vi "AuMT8852B EDR Differential Phase Encoding Configuration.vi"(5 "Settings":T1={"Low frequency selection"=enum."Use low frequency", "Medium frequency selection"=enum."Use medium frequency", "High frequency selection"=enum."Use high frequency", "Low TX frequency"=2480.0, "Medium TX frequency"=2402.0, "High TX frequency"=2402.0, "Percentage of packets limit"=99.0, "2DHx test packet"=enum."OFF", "3DHx test packet"=enum."OFF", "Hop selection"=enum."Test with hopping off and on", "Number of packets"=100} {"Percentage of packets limit" format="%.2f"}, 7 "Set/Get (Set)":enum16{"Set", "Get"}(ring), 8 "error in (no error)":errorcluster, 10 "Script (3)":i32=3, 11 "VISA session":refnum<visa-resource-name>) -> (0 "error out":errorcluster, 2 "error code":i32, 3 "VISA session out":refnum<visa-resource-name>, 4 "Settings out":T1={"Low frequency selection"=enum."Use low frequency", "Medium frequency selection"=enum."Use medium frequency", "High frequency selection"=enum."Use high frequency", "Low TX frequency"=2480.0, "Medium TX frequency"=2402.0, "High TX frequency"=2402.0, "Percentage of packets limit"=100.0, "2DHx test packet"=enum."OFF", "3DHx test packet"=enum."OFF", "Hop selection"=enum."Test with hopping off and on", "Number of packets"=7408} {"Percentage of packets limit" format="%.2f"})   [LabVIEW 2017]
doc: "Anritsu MT8852B Bluetooth Tester\n\nConfigures the instrument for the EDR Differential Phase Encoding test.\n\nINPUTS\nSet/Get - whether the values are being sent to or retrieved from the instrument.\nScript - which of the stored scripts (1-10) will be queried or configured. Scripts 1 and 2 are read-only.\nSettings - parameters of the test to be written.\n\nOUTPUTS\nSettings out - current parameters of the test."
uses:
  <instrlib>/aumt8852B/General/Utilities/MT8850 Test Parameters.ctl
  <instrlib>/aumt8852B/General/Utilities/MT8850 Frequency Units.ctl
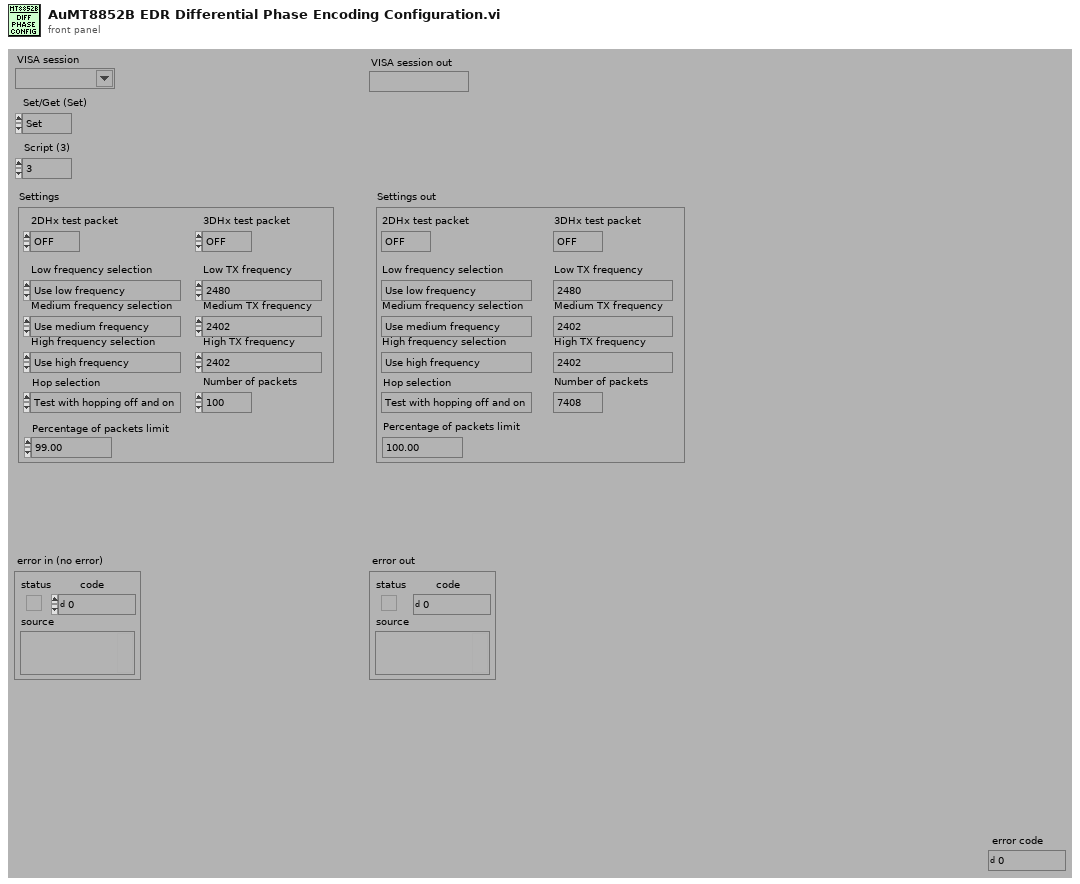
[diagram p1: front panel]
types:
  T1 = cluster{"Low frequency selection":enum16{"Don't use low frequency", "Use low frequency"}, "Medium frequency selection":enum16{"Don't use medium frequency", "Use medium frequency"}, "High frequency selection":enum16{"Don't use high frequency", "Use high frequency"}, "Low TX frequency":dbl, "Medium TX frequency":dbl, "High TX frequency":dbl, "Percentage of packets limit":dbl, "2DHx test packet":enum16{"OFF", "Longest", "2-DH1", "2-DH3", "2-DH5"}, "3DHx test packet":enum16{"OFF", "Longest", "3-DH1", "3-DH3", "3-DH5"}, "Hop selection":enum16{"Test with hopping on", "Test with hopping off", "Test with hopping off and on"}, "Number of packets":i32}
  T2 = enum16{"Output power", "Power control", "Modulation characteristics", "Initial carrier", "Carrier drift", "Single slot sensitivity", "Multiple slot sensitivity", "Maximum input power", "EDR Relative transmit power", "EDR Carrier frequency and stability", "EDR Differential phase encoding", "EDR Sensitivity", "EDR BER floor sensitivity", "EDR Maximum input power"}
  T3 = typedef "MT8850 Frequency Units.ctl" = enum16{"Channel", "Hz", "kHz", "MHz", "GHz"}
  T4 = typedef "MT8850 Test Parameters.ctl" = enum16{"Use low frequency", "Use medium frequency", "Use high frequency", "Low TX frequency", "Low RX frquency", "Medium TX frequency", "Medium RX frequency", "High TX frequency", "High RX frequency", "Number of packets", "Average high limit", "Average low limit", "Peak power limit", "Max power step limit", "Min power step limit", "f1 average minimum", "f1 average maximum", "f2 maximum", "f1/f2 average maximum", "Hop selection", "Use DH1 packets", "Use DH3 packets", "Use DH5 packets", "1 slot packet drift limit", "3 slot packet drift limit", "5 slot packet drift limit", "Drift rate limit", "TX power level", "Frequency offset", "Symbol timing", "Modulation index", "BER limit", "FER limit", "Use averaging high limit", "Use averaging low limit", "Use peak power limit", "Packet type", "Test control", "Use max power step limit", "Use min power step limit", "Number of cycles", "Use f1 average maximum", "Use f1 average minimum", "Use f2 maximum", "Use f1/f2 average maximum", "Hop mode", "Maximum negative limit", "Maximum positive limit", "Use maximum negative limit", "Use maximum positive limit", "Use 1 slot packet drift limit", "Use 3 slot packet drift limit", "Use 5 slot packet drift limit", "Use drift rate limit", "Use BER limit", "Use FER limit", "Use dirty parameter table", "Use null packet drift limit", "Null packet drift limit", "Minimum power", "Power delay", "Packet count", "Payload toggle", "Output power level", "2DHX packet type", "3DHX packet type", "Number of blocks", "TX and RX low frequency", "TX and RX medium frequency", "TX and RX high frequency", "TX frequency", "RX frequency", "Threshold bit count", "Total test bit count", "Number of bits", "PDPSK to PGFSK lower limit", "PDPSK to PGFSK upper limit", "Initial frequency error upper limit", "Initial frequency error lower limit", "Frequency error upper limit", "Frequency error lower limit", "Block frequency error upper limit", "Block frequency error lower limit", "2Mbs RMS DEVM limit", "3Mbs RMS DEVM limit", "2Mbs Peak DEVM limit", "3Mbs Peak DEVM limit", "2Mbs 99% packets DEVM limit", "3Mbs 99% packets DEVM limit", "Percentage of no error packets limit", "Threshold error limit", "Total test error limit"}
  T5 = enum16{"Simulate", "Range check", "Cache", "Query instrument status"}
  T6 = enum16{"Test with hopping on", "Test with hopping off", "Test with hopping off and on"}
  T7 = enum16{"OFF", "Longest", "3-DH1", "3-DH3", "3-DH5"}
  T8 = enum16{"OFF", "Longest", "2-DH1", "2-DH3", "2-DH5"}
  T9 = enum16{"Don't use high frequency", "Use high frequency"}
  T10 = enum16{"Don't use medium frequency", "Use medium frequency"}
  T11 = enum16{"Don't use low frequency", "Use low frequency"}
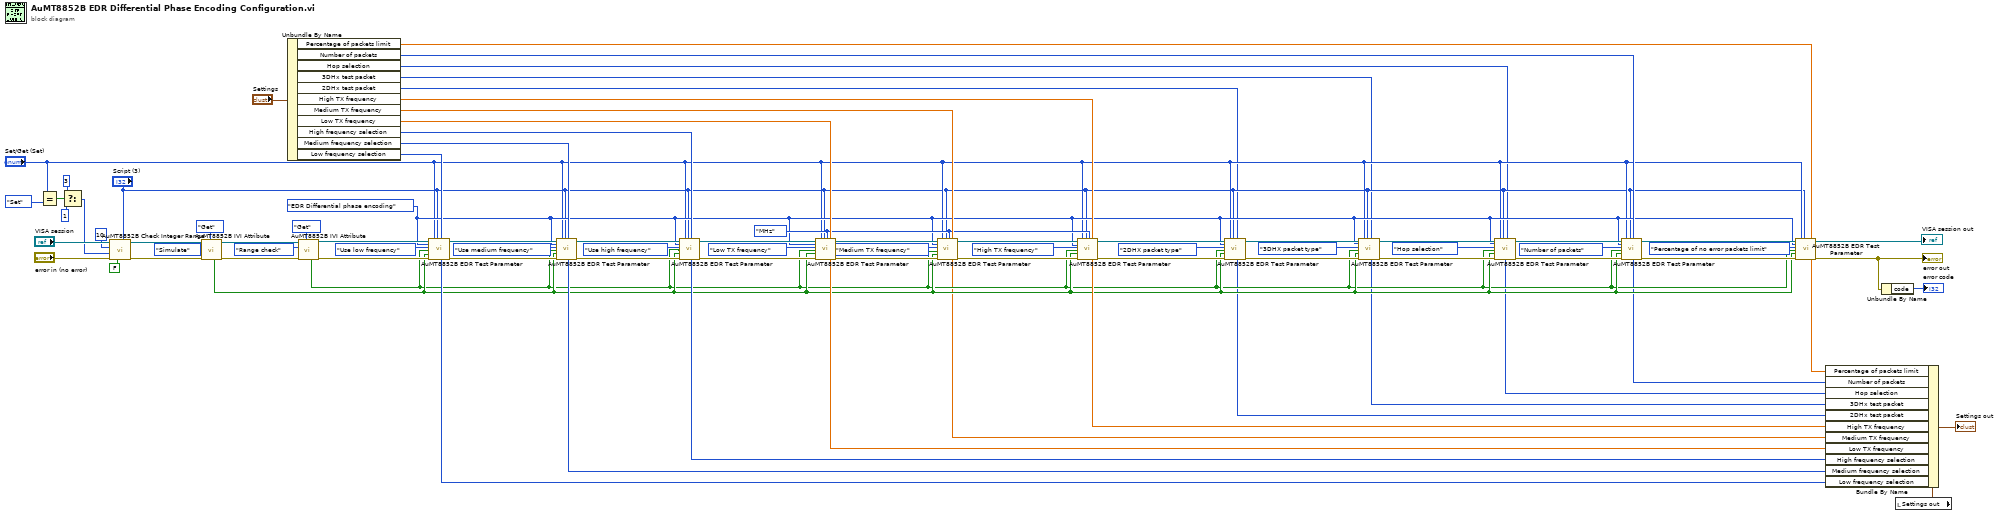
[diagram p0: block diagram]
diagram:
  w18 = T2."EDR Differential phase encoding" ("Test (Output power)")
  w19 = MT8850_Frequency_Units."MHz" ("Frequency units (MHz)")
  n1 = Equal?(x="Set/Get (Set)", y=enum16{"Set", "Get"}."Set") -> (x = y?=w81:bool)
  n2 = Select(t=3, s=w81, f=1) -> (s? t:f=w77:i32)
  n3 = call <instrlib>:"AuMT8852B Check Integer Range.vi"("Value (0)"="Script (3)", "Check IVI flag first? (T)"=FALSE, "error in (no error)"="error in (no error)", "Lower limit (-1)"=w77, "Upper limit (1)"=10, "VISA session"="VISA session") -> ("error out"=w75:errorcluster, "VISA session out"=w76:refnum<visa-resource-name>)  [unwired: 4 in]
  n4 = call <instrlib>:"AuMT8852B IVI Attribute.vi"("Set/Get (Set)"=enum16{"Set", "Get"}."Get", "error in (no error)"=w75, "Flag (Simulate)"=T5."Simulate", "VISA session"=w76) -> ("error out"=w49:errorcluster, "VISA session out"=w50:refnum<visa-resource-name>, "Value out"=w15:bool)  [unwired: 5 in]
  n5 = Unbundle By Name("Settings") -> ("Percentage of packets limit"=w30:dbl, "Number of packets"=w31:i32, "Hop selection"=w3:T6, "3DHx test packet"=w2:T7, "2DHx test packet"=w1:T8, "High TX frequency"=w38:dbl, "Medium TX frequency"=w39:dbl, "Low TX frequency"=w40:dbl, "High frequency selection"=w41:T9, "Medium frequency selection"=w42:T10, "Low frequency selection"=w43:T11)
  n6 = call <instrlib>:"AuMT8852B IVI Attribute.vi"("Set/Get (Set)"=enum16{"Set", "Get"}."Get", "error in (no error)"=w49, "Flag (Simulate)"=T5."Range check", "VISA session"=w50) -> ("error out"=w47:errorcluster, "VISA session out"=w48:refnum<visa-resource-name>, "Value out"=w14:bool)  [unwired: 5 in]
  n7 = call <instrlib>:"AuMT8852B EDR Test Parameter.vi"("VISA session"=w48, "Test (Output power)"=w18, "Parameter (Use low frequency)"=MT8850_Test_Parameters."Use low frequency", "Range check? (F)"=w14, "Simulate? (F)"=w15, "error in (no error)"=w47, "Set/Get (Set)"="Set/Get (Set)", "Script (3)"="Script (3)", "Integer value (0)"=w43) -> ("Integer value out"=w33:i32, "VISA session out"=w25:refnum<visa-resource-name>, "error out"=w24:errorcluster)  [unwired: 7 in, 1 out]
  n8 = call <instrlib>:"AuMT8852B EDR Test Parameter.vi"("VISA session"=w25, "Test (Output power)"=w18, "Parameter (Use low frequency)"=MT8850_Test_Parameters."Use medium frequency", "Range check? (F)"=w14, "Simulate? (F)"=w15, "error in (no error)"=w24, "Set/Get (Set)"="Set/Get (Set)", "Script (3)"="Script (3)", "Integer value (0)"=w42) -> ("Integer value out"=w34:i32, "VISA session out"=w23:refnum<visa-resource-name>, "error out"=w22:errorcluster)  [unwired: 7 in, 1 out]
  n9 = call <instrlib>:"AuMT8852B EDR Test Parameter.vi"("VISA session"=w23, "Test (Output power)"=w18, "Parameter (Use low frequency)"=MT8850_Test_Parameters."Use high frequency", "Range check? (F)"=w14, "Simulate? (F)"=w15, "error in (no error)"=w22, "Set/Get (Set)"="Set/Get (Set)", "Script (3)"="Script (3)", "Integer value (0)"=w41) -> ("Integer value out"=w35:i32, "VISA session out"=w71:refnum<visa-resource-name>, "error out"=w70:errorcluster)  [unwired: 7 in, 1 out]
  n10 = call <instrlib>:"AuMT8852B EDR Test Parameter.vi"("VISA session"=w71, "Test (Output power)"=w18, "Parameter (Use low frequency)"=MT8850_Test_Parameters."Low TX frequency", "Range check? (F)"=w14, "Simulate? (F)"=w15, "error in (no error)"=w70, "Set/Get (Set)"="Set/Get (Set)", "Script (3)"="Script (3)", "Integer value (0)"=w19, "Float value (0)"=w40) -> ("Float value out"=w36:dbl, "VISA session out"=w69:refnum<visa-resource-name>, "error out"=w68:errorcluster)  [unwired: 6 in, 1 out]
  n11 = call <instrlib>:"AuMT8852B EDR Test Parameter.vi"("VISA session"=w69, "Test (Output power)"=w18, "Parameter (Use low frequency)"=MT8850_Test_Parameters."Medium TX frequency", "Range check? (F)"=w14, "Simulate? (F)"=w15, "error in (no error)"=w68, "Set/Get (Set)"="Set/Get (Set)", "Script (3)"="Script (3)", "Integer value (0)"=w19, "Float value (0)"=w39) -> ("Float value out"=w13:dbl, "VISA session out"=w67:refnum<visa-resource-name>, "error out"=w66:errorcluster)  [unwired: 6 in, 1 out]
  n12 = call <instrlib>:"AuMT8852B EDR Test Parameter.vi"("VISA session"=w67, "Test (Output power)"=w18, "Parameter (Use low frequency)"=MT8850_Test_Parameters."High TX frequency", "Range check? (F)"=w14, "Simulate? (F)"=w15, "error in (no error)"=w66, "Set/Get (Set)"="Set/Get (Set)", "Script (3)"="Script (3)", "Integer value (0)"=w19, "Float value (0)"=w38) -> ("Float value out"=w37:dbl, "VISA session out"=w65:refnum<visa-resource-name>, "error out"=w64:errorcluster)  [unwired: 6 in, 1 out]
  n13 = call <instrlib>:"AuMT8852B EDR Test Parameter.vi"("VISA session"=w65, "Test (Output power)"=w18, "Parameter (Use low frequency)"=MT8850_Test_Parameters."2DHX packet type", "Range check? (F)"=w14, "Simulate? (F)"=w15, "error in (no error)"=w64, "Set/Get (Set)"="Set/Get (Set)", "Script (3)"="Script (3)", "Integer value (0)"=w1) -> ("Integer value out"=w12:i32, "VISA session out"=w63:refnum<visa-resource-name>, "error out"=w62:errorcluster)  [unwired: 7 in, 1 out]
  n14 = call <instrlib>:"AuMT8852B EDR Test Parameter.vi"("VISA session"=w63, "Test (Output power)"=w18, "Parameter (Use low frequency)"=MT8850_Test_Parameters."3DHX packet type", "Range check? (F)"=w14, "Simulate? (F)"=w15, "error in (no error)"=w62, "Set/Get (Set)"="Set/Get (Set)", "Script (3)"="Script (3)", "Integer value (0)"=w2) -> ("Integer value out"=w9:i32, "VISA session out"=w61:refnum<visa-resource-name>, "error out"=w60:errorcluster)  [unwired: 7 in, 1 out]
  n15 = call <instrlib>:"AuMT8852B EDR Test Parameter.vi"("VISA session"=w61, "Test (Output power)"=w18, "Parameter (Use low frequency)"=MT8850_Test_Parameters."Hop selection", "Range check? (F)"=w14, "Simulate? (F)"=w15, "error in (no error)"=w60, "Set/Get (Set)"="Set/Get (Set)", "Script (3)"="Script (3)", "Integer value (0)"=w3) -> ("Integer value out"=w11:i32, "VISA session out"=w59:refnum<visa-resource-name>, "error out"=w58:errorcluster)  [unwired: 7 in, 1 out]
  n16 = call <instrlib>:"AuMT8852B EDR Test Parameter.vi"("VISA session"=w59, "Test (Output power)"=w18, "Parameter (Use low frequency)"=MT8850_Test_Parameters."Number of packets", "Range check? (F)"=w14, "Simulate? (F)"=w15, "error in (no error)"=w58, "Set/Get (Set)"="Set/Get (Set)", "Script (3)"="Script (3)", "Integer value (0)"=w31) -> ("Integer value out"=w10:i32, "VISA session out"=w28:refnum<visa-resource-name>, "error out"=w27:errorcluster)  [unwired: 7 in, 1 out]
  n17 = call <instrlib>:"AuMT8852B EDR Test Parameter.vi"("VISA session"=w28, "Test (Output power)"=w18, "Parameter (Use low frequency)"=MT8850_Test_Parameters."Percentage of no error packets limit", "Range check? (F)"=w14, "Simulate? (F)"=w15, "error in (no error)"=w27, "Set/Get (Set)"="Set/Get (Set)", "Script (3)"="Script (3)", "Float value (0)"=w30) -> ("Float value out"=w8:dbl, "VISA session out"=→"VISA session out":refnum<visa-resource-name>, "error out"=w5:errorcluster)  [unwired: 7 in, 1 out]
  "error out" <- w5
  n18 = Unbundle By Name(w5) -> ("code"=→"error code":i32)
  n19 = local read "Settings out"() -> (w32:T1)
  n20 = Bundle By Name(cluster=w32, "Percentage of packets limit"=w8, "Number of packets"=w10, "Hop selection"=w11, "3DHx test packet"=w9, "2DHx test packet"=w12, "High TX frequency"=w37, "Medium TX frequency"=w13, "Low TX frequency"=w36, "High frequency selection"=w35, "Medium frequency selection"=w34, "Low frequency selection"=w33) -> (→"Settings out":T1)
